vi "Pot TBM.vi"(8 "error in":errorcluster, 10 "Slot":u32, 11 "SyringeTool in":refnum<class "SyringeTool Class.lvclass">) -> (0 "error out":errorcluster, 3 "SyringeTool out":refnum<class "SyringeTool Class.lvclass">)   [LabVIEW 2011, in "SyringeTool Class.lvclass"]
uses:
  SyringeTool Class.lvclass
  WorkTable Class/WorkTable Class.lvclass
  Vec3d Class/Vec3d Class.lvclass
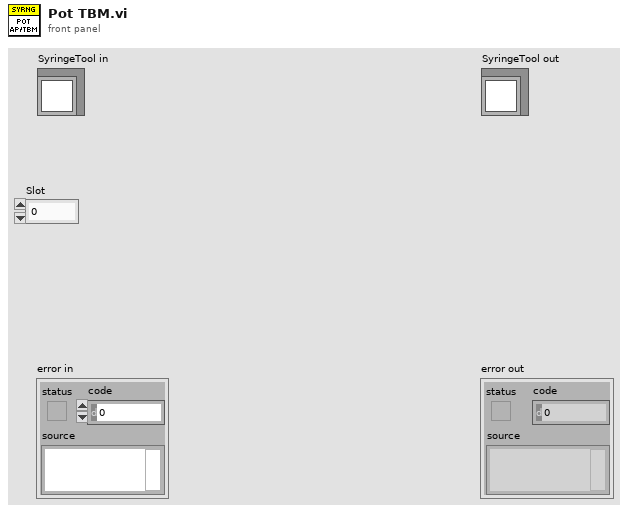
[diagram p1: front panel]
types:
  T1 = typedef "Worktable_HDI Slot.ctl" = cluster{"HDI Assembly State":enum16{"Empty", "Populated"}, "HDI Type":enum16{"HDI", "Polyimide"}, "Vacuum Channel":u32, "Location/Orientation":T2}
  T2 = typedef "Position_Orientation.ctl" = cluster{"Center":refnum<class "Vec3d Class.lvclass">, "Orientation":refnum<class "Orient3d Class.lvclass">}
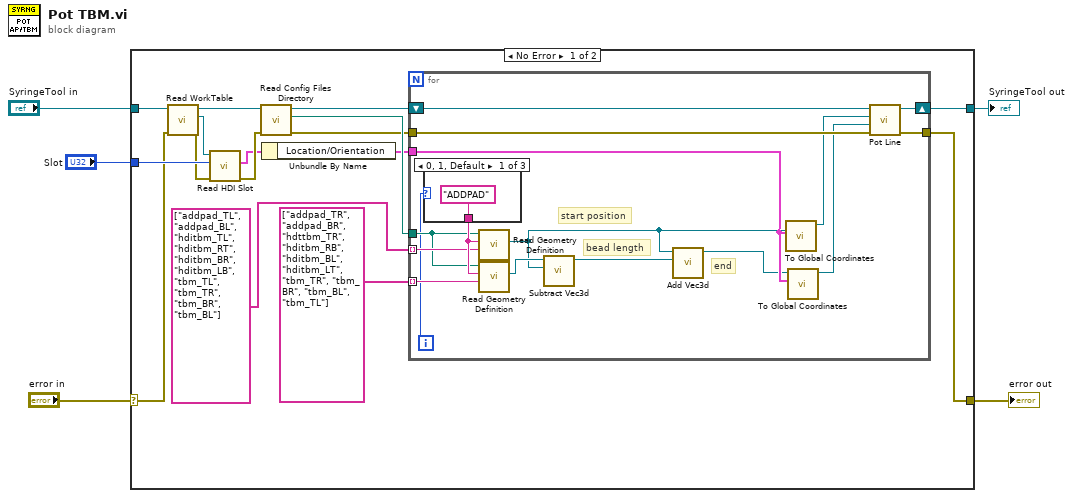
[diagram p0: block diagram]
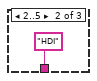
[diagram p2: hidden frame]
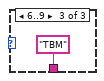
[diagram p3: hidden frame]
diagram:
  n1 = case shown="No Error" "error in" {
    selector: "error in" -> [w8 w42]
    tunnel: [w6 w42] -> w4
    tunnel: [w13 w41] -> w2
    tunnel: "SyringeTool in" -> [w21 w41]
    tunnel: "Slot" -> [w19 _]
    frame No Error {
      n2 = call-dynamic "Read WorkTable.vi"("error in"=w8, "Gantry Class in"=w21) -> ("error out"=w18:errorcluster, "WorkTable Class.lvclass"=w20:refnum<class "WorkTable Class.lvclass">, "Gantry Class out"=w17:refnum<class "SyringeTool Class.lvclass">)  [unwired: 7 in]
      n3 = call-dynamic "Read HDI Slot.vi"("error in"=w18, "HDI Slot Number"=w19, "WorkTable in"=w20) -> ("error out"=w16:errorcluster, "HDI Slot"=w15:T1)  [unwired: 6 in, 1 out]
      n4 = call-dynamic "Read Config Files Directory.vi"("error in (no error)"=w16, "Gantry Class in"=w17) -> ("error out"=w7:errorcluster, "Config Files Directory"=w11:path, "Gantry Class out"=w14:refnum<class "SyringeTool Class.lvclass">)  [unwired: 7 in]
      n5 = Unbundle By Name(w15) -> ("Location/Orientation"=w9:T2)
      n6 = for {
        shift-right: [w36] -> w13
        shift-left: w14 -> [w37]
        tunnel: string[] ["addpad_TR", "addpad_BR", "hdttbm_TR", "hditbm_RB", "hditbm_BL", "hditbm_LT", "tbm_TR", "tbm_BR", "tbm_BL", "tbm_TL"] -> [w33] mode=indexing
        tunnel: w11 -> [w31]
        tunnel: string[] ["addpad_TL", "addpad_BL", "hditbm_TL", "hditbm_RT", "hditbm_BR", "hditbm_LB", "tbm_TL", "tbm_TR", "tbm_BR", "tbm_BL"] -> [w32] mode=indexing
        tunnel: w9 -> [w28]
        tunnel: w7 -> [w27]
        tunnel: [w26] -> w6
        i -> [w22]
        # "end"
        # "start position"
        # "bead length"
        n7 = case shown="0, 1, Default" w22 {
          tunnel: ["ADDPAD" ("Part") "HDI" ("Part") "TBM" ("Part")] -> w35
          frame 0, 1, Default {
          }
          frame 2..5 {
          }
          frame 6..9 {
          }
        }
        n8 = call "Read Geometry Definition.vi"("Feature"=w32, "Part"=w35, "Config Location"=w31) -> ("Feature Coordinates"=w30:refnum<class "Vec3d Class.lvclass">)  [unwired: 7 in, 1 out]
        n9 = call "Read Geometry Definition.vi"("Feature"=w33, "Part"=w35, "Config Location"=w31) -> ("Feature Coordinates"=w34:refnum<class "Vec3d Class.lvclass">)  [unwired: 7 in, 1 out]
        n10 = call "Subtract Vec3d.vi"("Vec3d in 2"=w30, "Vec3d in 1"=w34) -> ("Vec3d Class out"=w29:refnum<class "Vec3d Class.lvclass">)  [unwired: 8 in, 1 out]
        n11 = call-dynamic "Add Vec3d.vi"(10:"Vec3d Class in"=w29, 11:"Vec3d Class in"=w30) -> ("Vec3d Class out"=w25:refnum<class "Vec3d Class.lvclass">)  [unwired: 8 in, 1 out]
        n12 = call "To Global Coordinates.vi"("Center/Orientation"=w28, "Local Coordinates"=w30) -> ("Global Coordinates"=w23:refnum<class "Vec3d Class.lvclass">)  [unwired: 8 in, 1 out]
        n13 = call "To Global Coordinates.vi"("Center/Orientation"=w28, "Local Coordinates"=w25) -> ("Global Coordinates"=w24:refnum<class "Vec3d Class.lvclass">)  [unwired: 8 in, 1 out]
        n14 = call-dynamic "Pot Line.vi"("error in"=w27, "End Position"=w24, "Start Position"=w23, "SyringeTool in"=w37) -> ("error out"=w26:errorcluster, "SyringeTool out"=w36:refnum<class "SyringeTool Class.lvclass">)  [unwired: 6 in]
      }
    }
    frame Error {
    }
  }
  "error out" <- w4
  "SyringeTool out" <- w2
